vi "ray_vector_to_element__v1.vi"(0 "光線ベクトル":ext[][](array[numeric])=[[0.0, 1.0], [2.0, 3.0], [4.0, 5.0]]) -> (14 "x":ext, 15 "α":ext=1.0, 16 "y":ext=2.0, 17 "β":ext=3.0, 18 "z":ext=4.0, 19 "γ":ext=5.0)   [LabVIEW 2020]
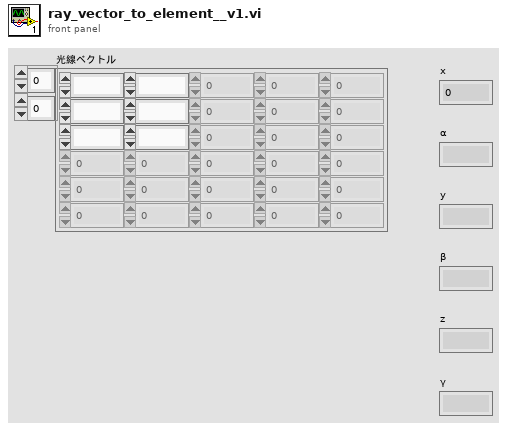
[diagram p1: front panel]
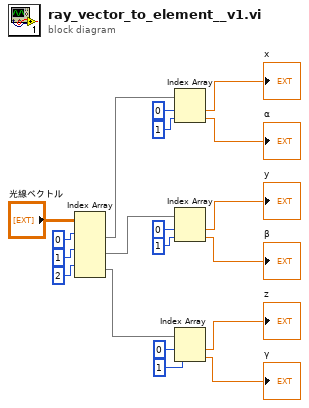
[diagram p0: block diagram]
diagram:
  n1 = Index Array(array="光線ベクトル", index (row) #1=0, index (row) #2=1, index (row) #3=2) -> (element #1=w15:ext[], element #2=w14:ext[], element #3=w13:ext[])  [unwired: 3 in]
  n2 = Index Array(array=w15, index #1=0, index #2=1) -> (element #1=→"x":ext, element #2=→"α":ext)
  n3 = Index Array(array=w14, index #1=0, index #2=1) -> (element #1=→"y":ext, element #2=→"β":ext)
  n4 = Index Array(array=w13, index #1=0, index #2=1) -> (element #1=→"z":ext, element #2=→"γ":ext)
